vi "Report.vi"(8 "error in (no error)":errorcluster, 11 "Pound":refnum<class "Pound.lvclass">) -> (0 "error out":errorcluster, 2 "Watchdog Report":T1(array[cluster]), 3 "Pound":refnum<class "Pound.lvclass">)   [LabVIEW 2017, in "Pound.lvclass"]
doc: "Reports the current status of each Watchdog associated with the Pound."
uses:
  <vilib>/NI/Software Watchdog/Pound/Pound.lvclass
  <vilib>/NI/Software Watchdog/Pound/Pound.lvclass/Pound.ctl
  <vilib>/NI/Software Watchdog/Watchdog/Watchdog.lvclass
  <vilib>/NI/Software Watchdog/Watchdog/Read MaxElapsedTime.vi
  <vilib>/NI/Software Watchdog/Watchdog/Read Timeout.vi
  <vilib>/NI/Software Watchdog/Watchdog/Read Name.vi
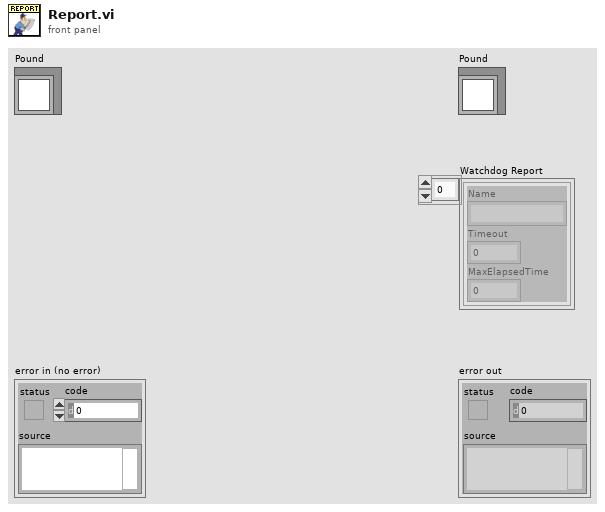
[diagram p1: front panel]
types:
  T1 = cluster{"Name":string, "Timeout":u32, "MaxElapsedTime":u32}[]
  T2 = cluster{"Name":string, "Execution Timeout":u32, "MaxElapsedTime":u32}
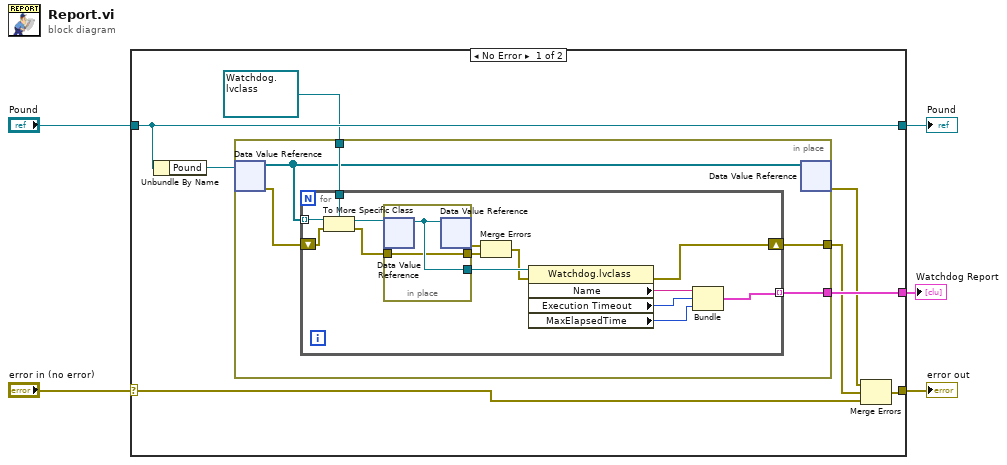
[diagram p0: block diagram]
diagram:
  n1 = case shown="No Error" "error in (no error)" {
    selector: "error in (no error)" -> [w6 w36]
    tunnel: [w9 w36] -> w4
    tunnel: [w13 w35] -> w2
    tunnel: "Pound" -> [w13 w35]
    tunnel: [w10 _] -> w1
    frame No Error {
      n2 = Unbundle By Name(w13) -> ("Pound"=w12:refnum<data-value>)
      n3 = in-place {
        in-place-border: refnum<data-value> refnum ("data value reference") -> [w17]
        in-place-border: [w15] -> w10
        in-place-border: [w14] -> w7
        n4 = in-place-dvr #1(w12) -> (w16:refnum<data-value>[], w18:errorcluster)
        n5 = for {
          tunnel: w16 -> [w32] mode=indexing
          tunnel: w17 -> [w30]
          tunnel: [w21] -> w15 mode=indexing
          shift-right: [w19] -> w14
          shift-left: w18 -> [w31]
          n6 = To More Specific Class(target class=w30, reference=w32, error in=w31) -> (specific class reference=w29:refnum<data-value>, error out=w28:errorcluster)
          n7 = in-place {
            in-place-border: w28 -> [w33]
            in-place-border: [w34] -> w22
            in-place-border: [w33] -> w26
            n8 = in-place-dvr #2(w29) -> (w34:refnum<class "Watchdog.lvclass">)  [unwired: 1 out]
            n9 = in-place-dvr #2(w34) -> (w27:errorcluster)  [unwired: 1 out]
          }
          n10 = Merge Errors(w27, w26) -> (w20:errorcluster)
          n11 = property class="Watchdog.lvclass"(reference=w22, error in=w20) -> (error out=w19:errorcluster, "Name"=w25:string, "Execution Timeout"=w24:u32, "MaxElapsedTime"=w23:u32)  [unwired: 1 out]
          n12 = Bundle("Name"=w25, "Execution Timeout"=w24, "MaxElapsedTime"=w23) -> (w21:T2)  [unwired: 1 in]
        }
        n13 = in-place-dvr #1(w16) -> (w8:errorcluster)  [unwired: 1 out]
      }
      n14 = Merge Errors(w8, w7, w6) -> (w9:errorcluster)
    }
    frame Error {
    }
  }
  "error out" <- w4
  "Pound" <- w2
  "Watchdog Report" <- w1
